vi "AcquireHardware.vi"(8 "error in (no error)":errorcluster, 11 "Point Grey Camera in":refnum<class "Point Grey Camera.lvclass">) -> (0 "error out":errorcluster, 2 "Image Out":T1(plugin-control), 3 "Point Grey Camera out":refnum<class "Point Grey Camera.lvclass">)   [LabVIEW 2020, in "Point Grey Camera.lvclass"]
uses:
  Point Grey Camera.lvclass
  Point Grey Camera.lvclass/Point Grey Camera.ctl
  NI_Vision_Acquisition_Software.lvlib
  NI_Vision_Development_Module.lvlib
  <resource>/objmgr/imaqdx.rc
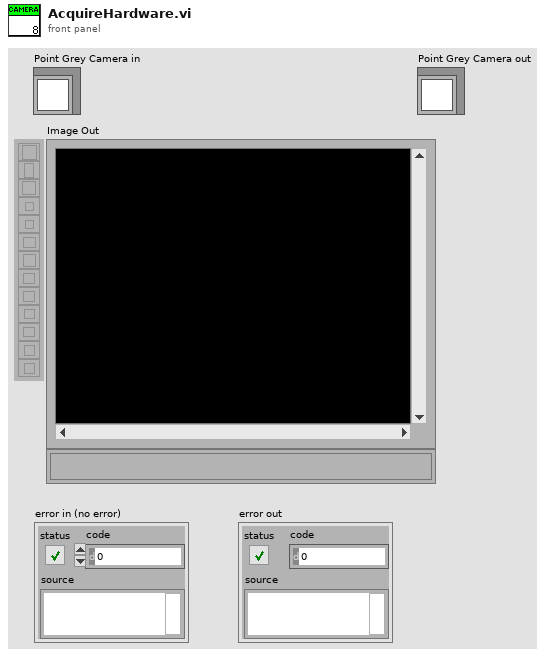
[diagram p1: front panel]
types:
  T1 = typedef "IMAQ Image.ctl" = refnum<image>
  T2 = typedef "IMAQdx.ctl" = refnum<k21>
  T3 = typedef "OnOffTypeDef.ctl" = enum16{"off", "on"}
  T4 = typedef "Image Type" = u32
  T5 = cluster{"histogram":u32[], "Minimal Value":sgl, "Maximal Value":sgl, "Starting Value":sgl, "Interval Width":sgl, "Mean Value":sgl, "Standard  Variation":sgl, "Area (pixels)":i32}
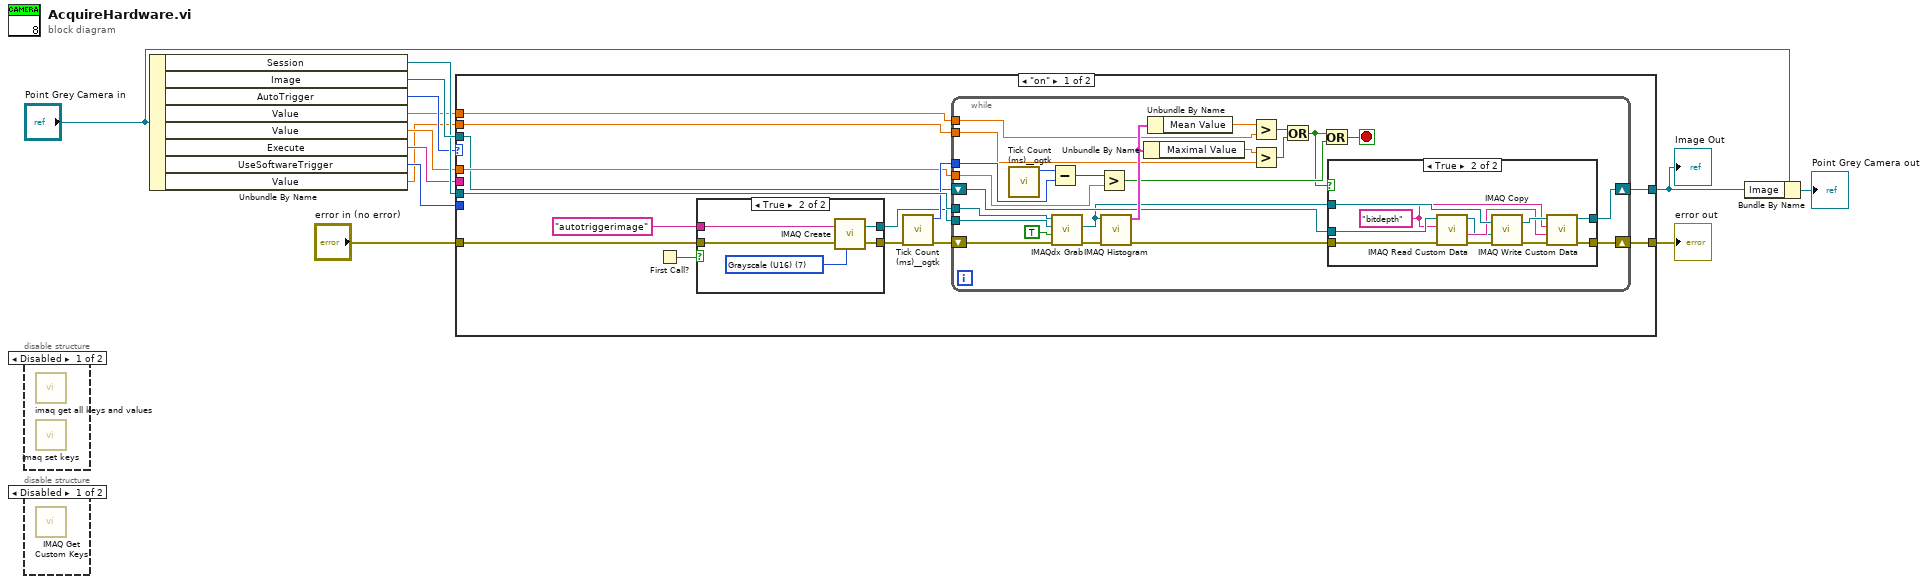
[diagram p0: block diagram]
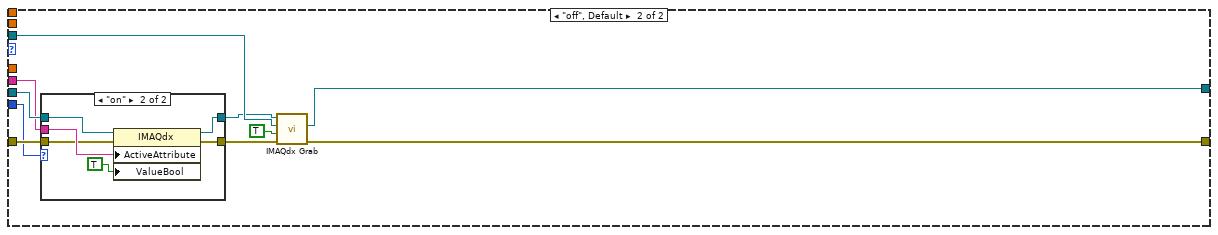
[diagram p6: hidden frame]
diagram:
  n1 = disable-structure shown="Disabled" {
    frame Disabled {
      n2 = call "imaq get all keys and values.vi"() -> ()  [unwired: 8 in, 4 out]
      n3 = call "imaq set keys.vi"() -> ()  [unwired: 10 in, 2 out]
    }
    frame Enabled {
    }
  }
  n4 = disable-structure shown="Disabled" {
    frame Disabled {
      n5 = call "IMAQ Get Custom Keys"() -> ()  [unwired: 8 in, 4 out]
    }
    frame Enabled {
    }
  }
  n6 = Unbundle By Name("Point Grey Camera in") -> ("Session"=w12:T2, "Image"=w13:T1, "AutoTrigger"=w8:T3, "Value"=w7:dbl, "Value"=w6:dbl, "Execute"=w3:string, "UseSoftwareTrigger"=w2:T3, "Value"=w1:dbl)
  n7 = case shown="\"on\"" w8 {
    tunnel: w13 -> [w17 w81]
    tunnel: w12 -> [w27 w77]
    tunnel: [w26 w80] -> w4
    tunnel: "error in (no error)" -> [w16 w75]
    tunnel: [w25 w78] -> w9
    tunnel: w7 -> [w22 _]
    tunnel: w6 -> [w21 _]
    tunnel: w3 -> [_ w76]
    tunnel: w2 -> [_ w72]
    tunnel: w1 -> [w14 _]
    frame "on" {
      n8 = First Call?() -> (First Call?: T/F=w20:bool)
      n9 = case shown="True" w20 {
        tunnel: [w29 w34] -> w19
        tunnel: "autotriggerimage" ("Image Name") -> [w29 w33]
        tunnel: w16 -> [w28 w31]
        tunnel: [w28 w30] -> w15
        frame False {
        }
        frame True {
          w32 = T4 7 items=["Grayscale (U8)", "Grayscale (I16)", "Grayscale (SGL)", "Complex (CSG)", "RGB (U32)", "HSL (U32)", "RGB (U64)", "Grayscale (U16)"] ("Image Type")
          n10 = call "IMAQ Create"("Image Name"=w33, "Image Type"=w32, "error in (no error)"=w31) -> ("New Image"=w34:T1, "error out"=w30:errorcluster)  [unwired: 2 in]
        }
      }
      n11 = call "Tick Count (ms)__ogtk.vi"("error in (no error)"=w15) -> ("error out"=w24:errorcluster, "millisecond timer value"=w23:u32)  [unwired: 9 in]
      n12 = while {
        tunnel: w27 -> [w58]
        shift-right: [w45] -> w25
        shift-left: w17 -> [w46]
        shift-right: [w43] -> w26
        shift-left: w24 -> [w57]
        tunnel: w23 -> [w52]
        tunnel: w22 -> [w49]
        tunnel: w21 -> [w48]
        tunnel: w19 -> [w47]
        tunnel: w14 -> [w39]
        stop <- w54 stop-if-true
        n13 = call "Tick Count (ms)__ogtk.vi"() -> ("millisecond timer value"=w53:u32)  [unwired: 10 in, 1 out]
        n14 = Subtract(x=w53, y=w52) -> (x-y=w51:u32)
        n15 = call "IMAQdx Grab.vi"("error in"=w57, "Wait for Next Buffer? (Yes)"=TRUE, "Image In"=w47, "Session In"=w58) -> ("error out"=w41:errorcluster, "Image Out"=w42:T1)  [unwired: 6 out]
        n16 = Greater?(x=w51, y=w48) -> (0:w50:bool)
        n17 = call "IMAQ Histogram"("error in (no error)"=w41, "Image"=w42) -> ("error out"=w44:errorcluster, "Histogram Report"=w55:T5)  [unwired: 8 in]
        n18 = Unbundle By Name(w55) -> ("Maximal Value"=w38:sgl)
        n19 = Unbundle By Name(w55) -> ("Mean Value"=w40:sgl)
        n20 = Greater?(x=w40, y=w49) -> (0:w37:bool)
        n21 = Greater?(x=w38, y=w39) -> (0:w36:bool)
        n22 = Or(x=w37, y=w36) -> (x .or. y?=w35:bool)
        n23 = Or(x=w35, y=w50) -> (x .or. y?=w54:bool)
        n24 = case shown="True" w35 {
          tunnel: w42 -> [_ w71]
          tunnel: w46 -> [w60 w69]
          tunnel: [w60 w61] -> w45
          tunnel: w44 -> [w59 w65]
          tunnel: [w59 w62] -> w43
          frame False {
          }
          frame True {
            w68 = "bitdepth" ("Key")
            n25 = call "IMAQ Read Custom Data"("error in (no error)"=w65, "Key"=w68, "Image"=w69) -> ("error out"=w64:errorcluster, "Custom Data Out"=w67:string, "Image (duplicate)"=w66:T1)  [unwired: 6 in]
            n26 = call "IMAQ Copy"("error in (no error)"=w64, "Image Dst"=w66, "Image Src"=w71) -> ("error out"=w63:errorcluster, "Image Dst Out"=w70:T1)  [unwired: 3 in]
            n27 = call "IMAQ Write Custom Data"("error in (no error)"=w63, "Custom Data In"=w67, "Key"=w68, "Image"=w70) -> ("error out"=w62:errorcluster, "Image Out"=w61:T1)  [unwired: 6 in]
          }
        }
      }
    }
    frame "off", Default {
      n28 = case shown="\"on\"" w72 {
        tunnel: w77 -> [w83 w89]
        tunnel: w76 -> [_ w88]
        tunnel: w75 -> [w82 w86]
        tunnel: [w82 w85] -> w74
        tunnel: [w83 w84] -> w73
        frame "off", Default {
        }
        frame "on" {
          n29 = property class="IMAQdx"(reference=w89, error in=w86, "ActiveAttribute"=w88, "ValueBool"=TRUE) -> (reference out=w84:T2, error out=w85:errorcluster)
        }
      }
      n30 = call "IMAQdx Grab.vi"("error in"=w74, "Wait for Next Buffer? (Yes)"=TRUE, "Image In"=w81, "Session In"=w73) -> ("error out"=w80:errorcluster, "Image Out"=w78:T1)  [unwired: 6 out]
    }
  }
  "Image Out" <- w9
  "error out" <- w4
  n31 = Bundle By Name(cluster="Point Grey Camera in", "Image"=w9) -> (→"Point Grey Camera out":refnum<class "Point Grey Camera.lvclass">)
